vi "Calibrate.vi"(8 "error in (no error)":errorcluster, 11 "Instrument in":refnum<class "Test Instrument.lvclass">) -> (0 "error out":errorcluster, 1 "Success?":bool, 2 "Result":variant, 3 "Instrument out":refnum<class "Test Instrument.lvclass">)   [LabVIEW 2020, in "Test.lvlib" / "Test Instrument.lvclass"]
doc: "Calibrate the instrument if supported. The calibration result is returned in a variant.\n\nThe default implementation does nothing."
uses:
  Test Instrument.lvclass
  PPL/HDH.Actor Framework.Core.Instrument Driver.lvlibp/Instrument Driver/Instrument Driver.lvclass
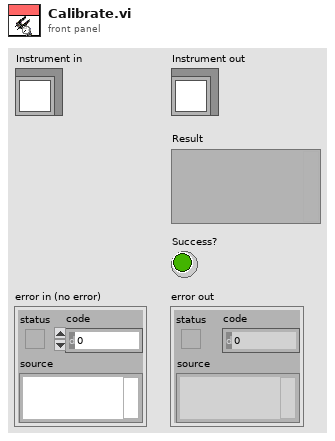
[diagram p1: front panel]
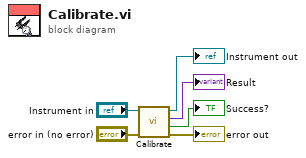
[diagram p0: block diagram]
diagram:
  n1 = call-parent "Calibrate.vi"("error in (no error)"="error in (no error)", "Instrument in"="Instrument in") -> ("error out"=→"error out":errorcluster, "Success?"=→"Success?":bool, "Result"=→"Result":variant, "Instrument out"=→"Instrument out":refnum<class "Test Instrument.lvclass">)  [unwired: 6 in]
